vi "HT I2C Config.vi"(9 "error in (no error)":errorcluster, 11 "Channel Name":tag="A/I2C") -> (0 "error out":errorcluster, 2 "I2C Ref Out":T1)   [LabVIEW 2017]
uses:
  <vilib>/myRIO/Instrument Drivers/Onboard IO/I2C/typedefs/I2C Reference.ctl
  <vilib>/myRIO/Common/Instrument Driver Framework/Utilities/typedefs/myRIO Generic Hardware Reference.ctl
  <vilib>/myRIO/Common/Instrument Driver Framework/Utilities/typedefs/Hardware Version Enum.ctl
  <vilib>/myRIO/Common/Instrument Driver Framework/Utilities/typedefs/myRIO v1.0 Reference.ctl
  <vilib>/myRIO/Common/Instrument Driver Framework/Utilities/typedefs/Generic FPGA Reference.ctl
  <vilib>/myRIO/Common/Instrument Driver Framework/myRIO v1.0/I2C/typedefs/I2C Channels Enum.ctl
  <vilib>/myRIO/Instrument Drivers/Onboard IO/I2C/typedefs/I2C Configuration.ctl
  <vilib>/myRIO/Instrument Drivers/Onboard IO/I2C/typedefs/I2C Transfer Rate.ctl
  <vilib>/myRIO/Instrument Drivers/Onboard IO/I2C/typedefs/I2C User Configuration.ctl
  <vilib>/Utility/error.llb/Error Cluster From Error Code.vi
  <vilib>/myRIO/Common/Instrument Driver Framework/myRIO v1.0/I2C/vis/myRIO v1.0 Configure I2C.vi
  <vilib>/myRIO/Instrument Drivers/Onboard IO/I2C/I2C.lvlib
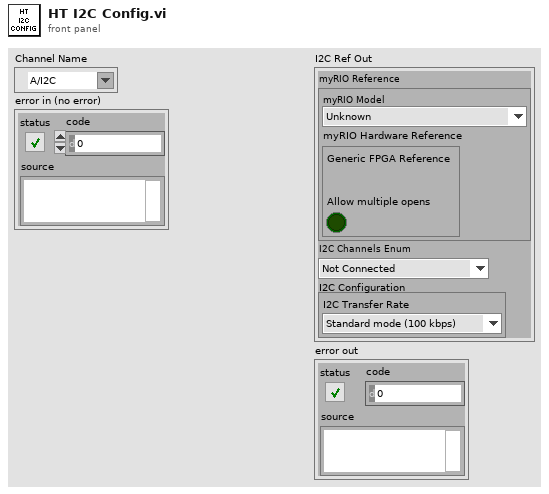
[diagram p1: front panel]
types:
  T1 = typedef "I2C.lvlib/I2C Reference.ctl" = cluster{"myRIO Reference":T2, "I2C Channels Enum":T6, "I2C Configuration":T7}
  T2 = typedef "myRIO Generic Hardware Reference.ctl" = cluster{"myRIO Model":T3, "myRIO Hardware Reference":T4}
  T3 = typedef "Hardware Version Enum.ctl" = enum16{"Unknown", "myRIO-1900", "myRIO-1950", "roboRIO", "NI ELVIS RIO CM"}
  T4 = typedef "myRIO v1.0 Reference.ctl" = cluster{"Generic FPGA Reference":T5, "Allow multiple opens":bool}
  T5 = typedef "Generic FPGA Reference.ctl" = refnum<k20>
  T6 = typedef "I2C Channels Enum.ctl" = enum16{"Not Connected", "A/I2C", "B/I2C", "I2C/I2C"}
  T7 = typedef "I2C.lvlib/I2C Configuration.ctl" = cluster{"I2C Transfer Rate":T8}
  T8 = typedef "I2C.lvlib/I2C Transfer Rate.ctl" = enum16{"Standard mode (100 kbps)", "Fast mode (400 kbps)"}
  T9 = typedef "I2C.lvlib/I2C User Configuration.ctl" = cluster{"I2C Transfer Rate":T8}
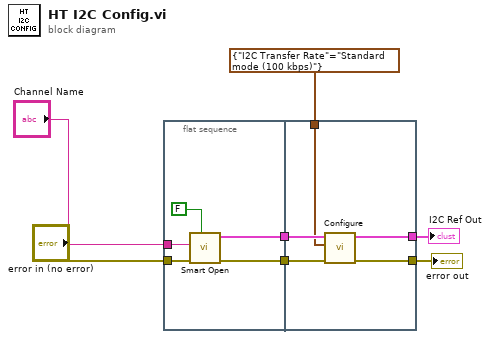
[diagram p0: block diagram]
diagram:
  n1 = flat-sequence {
    tunnel: "Channel Name" -> [w11]
    tunnel: "error in (no error)" -> [w10]
    tunnel: [w9] -> w5
    tunnel: [w8] -> w4
    tunnel: w5 -> [w17]
    tunnel: w4 -> [w16]
    tunnel: T9 {"I2C Transfer Rate"=enum."Standard mode (100 kbps)"} ("I2C User Configuration") -> [w15]
    tunnel: [w14] -> w2
    tunnel: [w13] -> w1
    frame #0 {
      n2 = call <vilib>:"Smart Open.vi"("Allow multiple opens?"=FALSE, "error in (no error)"=w10, "Channel Name"=w11) -> ("error out"=w8:errorcluster, "I2C Ref Out"=w9:T1)  [unwired: 7 in]
    }
    frame #1 {
      n3 = call <vilib>:"Configure.vi"("error in (no error)"=w16, "I2C User Configuration"=w15, "I2C Ref In"=w17) -> ("error out"=w13:errorcluster, "I2C Ref Out"=w14:T1)  [unwired: 7 in]
    }
  }
  "I2C Ref Out" <- w2
  "error out" <- w1
